vi "Result.vi"(8 "error in (no error)":errorcluster, 10 "Result":T1={"Name"="", "Description"="", "Status"=enum."Passed", "Result Type"=enum."Test Suite", "Execution Time"=0.0, "Data"={"Expected"=variant, "Actual"=variant, "Delta"=variant}}, 11 "XML Report In":refnum<class "XML Report.lvclass">) -> (0 "error out":errorcluster, 3 "XML Report Out":refnum<class "XML Report.lvclass">)   [LabVIEW 2020, in "XML Report.lvclass"]
uses:
  XML Report.lvclass
  Core/Result/Result.ctl
  Core/Result/Status.ctl
  Core/Result/Type.ctl
  XML Report.lvclass/XML Report.ctl
  Case Result.ctl
  <vilib>/Utility/miscctls.llb/LVMapReplaceAction.ctl
  Core/Result/Result.lvlib
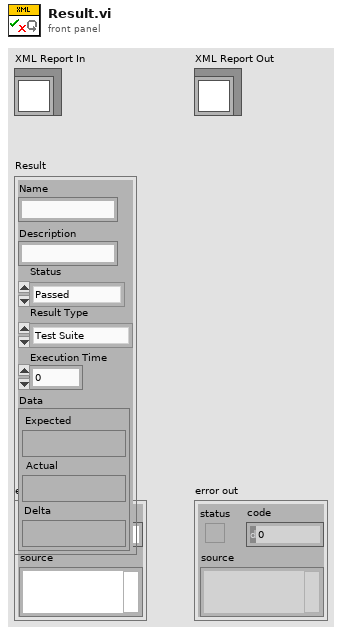
[diagram p1: front panel]
types:
  T1 = typedef "Result.lvlib/Result.ctl" = cluster{"Name":string, "Description":string, "Status":T2, "Result Type":T3, "Execution Time":dbl, "Data":cluster{"Expected":variant, "Actual":variant, "Delta":variant}}
  T2 = typedef "Result.lvlib/Status.ctl" = enum16{"", "Passed", "Failed", "Error", "Skipped", "Setup Error", "Broken", "Teardown Error"}
  T3 = typedef "Result.lvlib/Type.ctl" = enum16{"Test Case", "Test Suite", "Test Run", "Pass", "Fail", "Skip", "Pass if", "Fail if", "Pass if Error", "Fail if Error", "Pass if Equal", "Fail if Equal"}
  T4 = typedef "XML Report.lvclass/Case Result.ctl" = cluster{"Name":string, "Assertions":i32, "Classname":string, "Status":T2, "Time":dbl}
  T5 = typedef "LVMapReplaceAction.ctl" = enum32{"Modify Entry only if found", "Add or Modify Entry", "Delete Entry"}
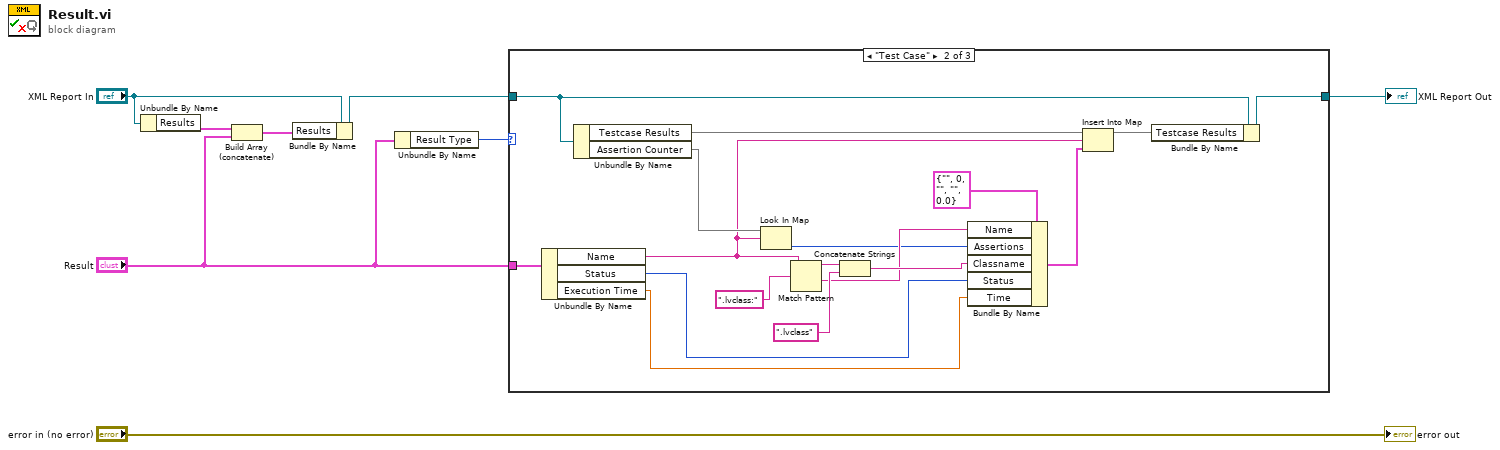
[diagram p0: block diagram]
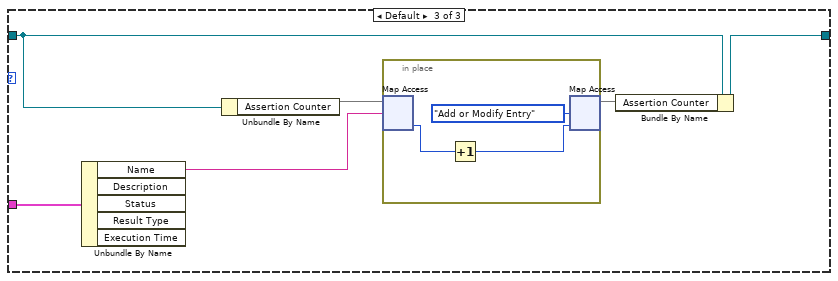
[diagram p3: hidden frame]
diagram:
  n1 = Unbundle By Name("XML Report In") -> ("Results"=w4:T1[])
  n2 = Build Array (concatenate)(w4, "Result") -> (w2:T1[])
  n3 = Bundle By Name(cluster="XML Report In", "Results"=w2) -> (w3:refnum<class "XML Report.lvclass">)
  n4 = Unbundle By Name("Result") -> ("Result Type"=w6:T3)
  n5 = case shown="\"Test Case\"" w6 {
    tunnel: w3 -> [w9 w23 w28]
    tunnel: [w9 w22 w32] -> w7
    tunnel: "Result" -> [_ w26 w27]
    frame "Test Run" {
    }
    frame "Test Case" {
      n6 = Unbundle By Name(w26) -> ("Name"=w13:string, "Status"=w11:T2, "Execution Time"=w10:dbl)
      n7 = Unbundle By Name(w23) -> ("Testcase Results"=w21:map{string, T4}, "Assertion Counter"=w14:map{string, i32})
      n8 = Look In Map(map=w14, key=w13) -> (value=w12:i32)  [unwired: 1 in, 1 out]
      n9 = Match Pattern(string=w13, regular expression=".lvclass:") -> (before substring=w24:string, after substring=w15:string)  [unwired: 1 in, 2 out]
      n10 = Concatenate Strings(w24, ".lvclass" ("string")) -> (w16:string)
      n11 = Bundle By Name(cluster=T4 {"Name"="", "Assertions"=0, "Classname"="", "Status"=enum."", "Time"=0.0} ("value"), "Name"=w15, "Assertions"=w12, "Classname"=w16, "Status"=w11, "Time"=w10) -> (w18:T4)
      n12 = Insert Into Map(map in=w21, key=w13, value=w18) -> (map out=w20:map{string, T4})  [unwired: 2 out]
      n13 = Bundle By Name(cluster=w23, "Testcase Results"=w20) -> (w22:refnum<class "XML Report.lvclass">)
    }
    frame Default {
      n14 = Unbundle By Name(w27) -> ("Name"=w29:string)  [unwired: 4 out]
      n15 = Unbundle By Name(w28) -> ("Assertion Counter"=w31:map{string, i32})
      n16 = in-place {
        n17 = in-place-map #1(w31, w29) -> (w34:i32)  [unwired: 1 in, 1 out]
        n18 = Increment(x=w34) -> (x+1=w33:i32)
        n19 = in-place-map #1(w33, LVMapReplaceAction."Add or Modify Entry" ("action")) -> (w30:map{string, i32})  [unwired: 2 out]
      }
      n20 = Bundle By Name(cluster=w28, "Assertion Counter"=w30) -> (w32:refnum<class "XML Report.lvclass">)
    }
  }
  "XML Report Out" <- w7
  "error out" <- "error in (no error)"
